vi "Assert Warning.vi"(4 "Execution time (s)":dbl=-1.0, 6 "error code (1)":i32=1, 7 "Label":string, 8 "error in":errorcluster, 11 "warning":errorcluster) -> (0 "error out":errorcluster, 2 "Properties":refnum<class "Properties.Assert.lvclass">)   [LabVIEW 2021, in "Banana.Caraya.lvlib" / "Platano.CarayaTestSuite.lvclass"]
uses:
  Platano.CarayaTestSuite.lvclass
  Platano.CarayaTestSuite.lvclass/Platano.CarayaTestSuite.ctl
  <vilib>/addons/_JKI Toolkits/Caraya/classes/Assert/Assert.lvclass
  Bananas/Platano/Platano.lvclass
  Bananas/Banana/Banana.lvclass
  <vilib>/addons/_JKI Toolkits/Caraya/classes/Assert/Assert True.vi
  Leaf.Properties.Assert/Leaf.Properties.Assert.lvclass
  Bananas/Leaf/Leaf.lvclass
  C:/Repositories/LVOS/Bananas/lv-src/Banana.Caraya/Leaf.Properties/Leaf.Properties.lvclass
  C:/Program Files (x86)/National Instruments/LabVIEW 2021/vi.lib/addons/_JKI Toolkits/Caraya/classes/Properties/Properties.lvclass
  C:/Repositories/LVOS/Bananas/lv-src/Bananas/Leaf.Assertion/Leaf.Assertion.lvclass
  C:/Repositories/LVOS/Bananas/lv-src/Bananas/Leaf/Leaf.lvclass
  C:/Repositories/LVOS/Bananas/lv-src/Banana.Caraya/Leaf.Properties.Assert/Leaf.Properties.Assert.lvclass
  Bananas/AssetError/AssertError.lvclass
  C:/Repositories/LVOS/Bananas/lv-src/Bananas/AssetError/AssertError.lvclass
  C:/Repositories/LVOS/Bananas/lv-src/Bananas/BananaPeel/BananaPeel.lvclass
  Bananas/Leaf.Assertion/Leaf.Assertion.lvclass
  <vilib>/addons/_JKI Toolkits/Caraya/classes/Properties.Assert/Properties.Assert.lvclass
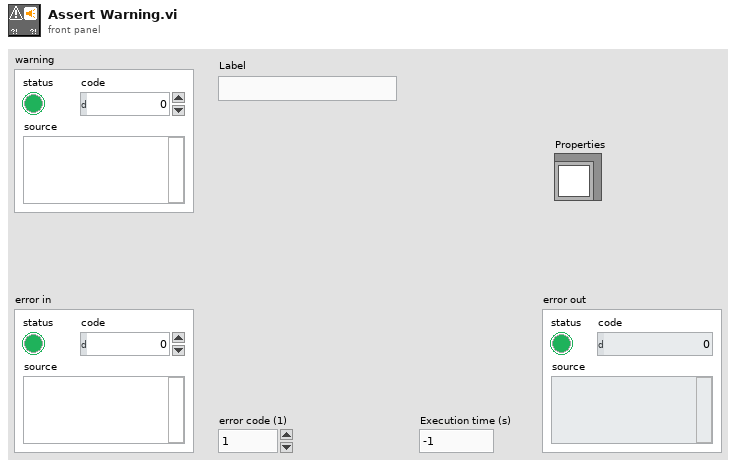
[diagram p1: front panel]
types:
  T1 = typedef "Bananas.lvlib/Assertion Strategies -- cluster.ctl" = cluster{"AssertTrue":refnum<class "AssertTrue.lvclass">, "AssertFalse":refnum<class "AssertFalse.lvclass">, "AssertEqualValue":refnum<class "AssertEqualValue.lvclass">, "AssertEqualType":refnum<class "AssertEqualType.lvclass">, "AssertCompareValue":refnum<class "AssertCompareValue.lvclass">, "AssertError":refnum<class "AssertError.lvclass">, "AssertAlmostEqual":refnum<class "AssertAlmostEqualValue.lvclass">}
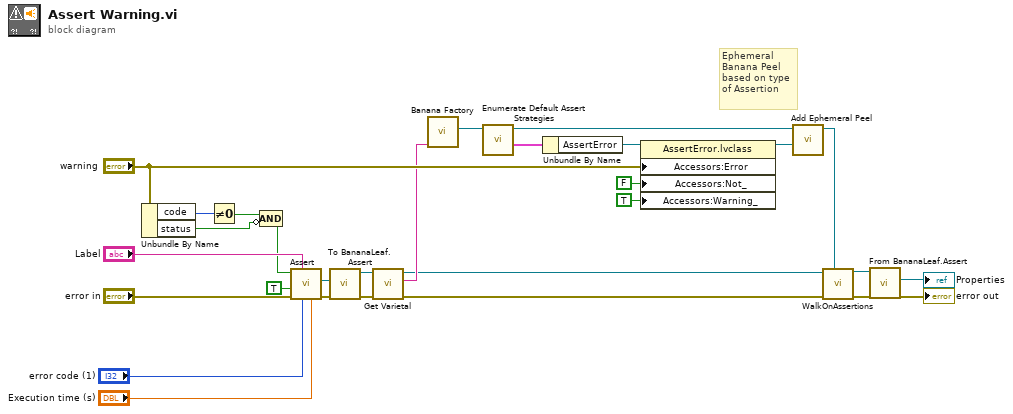
[diagram p0: block diagram]
diagram:
  # "Ephemeral\nBanana Peel\nbased on type\nof Assertion"
  n1 = Unbundle By Name("warning") -> ("code"=w13:i32, "status"=w11:bool)
  n2 = Not Equal To 0?(x=w13) -> (x != 0?=w12:bool)
  n3 = Compound Arithmetic op=AND(w12, invert w11) -> (w10:bool)
  n4 = call-poly <vilib>:"Assert.vi"("Execution time (s)"="Execution time (s)", "error code (1)"="error code (1)", "Label"="Label", "error in (no error)"="error in", "Register with caller test (F)"=TRUE, "True?"=w10) -> ("error out"=w5:errorcluster, "Properties"=w7:refnum<class "Properties.Assert.lvclass">)  [unwired: 4 in]
  n5 = call "To BananaLeaf.Assert.vi"("Properties.Assert"=w7) -> ("Leaf.Properties.Assert out"=w8:refnum<class "Leaf.Properties.Assert.lvclass">)  [unwired: 10 in]
  n6 = call "Get Varietal.vi"("error in (no error)"=w5, "Leaf in"=w8) -> ("error out"=w6:errorcluster, "Varietal"=w4:string, "Leaf out"=w3:refnum<class "Leaf.Properties.Assert.lvclass">)  [unwired: 7 in]
  n7 = call "Banana Factory.vi"("Varietal"=w4) -> ("Banana"=w9:refnum<class "Banana.lvclass">)  [unwired: 9 in, 1 out]
  n8 = call "Enumerate Default Assert Strategies.vi"("Banana"=w9) -> ("Strategies"=w19:T1, "Banana"=w20:refnum<class "Banana.lvclass">)  [unwired: 9 in]
  n9 = Unbundle By Name(w19) -> ("AssertError"=w18:refnum<class "AssertError.lvclass">)
  n10 = property class="AssertError.lvclass"(reference=w18, "Accessors:Error"="warning", "Accessors:Not_"=FALSE ("Not_"), "Accessors:Warning_"=TRUE ("Warning_")) -> (reference out=w17:refnum<class "AssertError.lvclass">)  [unwired: 1 in, 1 out]
  n11 = call "Add Ephemeral Peel.vi"("BananaPeel"=w17, "Banana"=w20) -> ("Banana"=w21:refnum<class "Banana.lvclass">)  [unwired: 9 in]
  n12 = call "WalkOnAssertions.vi"("Banana"=w21, "error in (no error)"=w6, "Leaf.Assertion"=w3) -> ("error out"=→"error out":errorcluster, "Leaf.Assertion"=w2:refnum<class "Leaf.Assertion.lvclass">)  [unwired: 7 in]
  n13 = call "From BananaLeaf.Assert.vi"("Leaf.Properties.Assert"=w2) -> ("Properties.Assert"=→"Properties":refnum<class "Properties.Assert.lvclass">)  [unwired: 10 in]
